vi "SwerveShortestTurnAlg.vi"(7 "Joystick Axes":dbl[](array[numeric]), 8 "SwerveMotorsFlipped?":bool, 9 "SwerveSpeed":dbl, 10 "AngleSetpoint":dbl, 11 "AngleEncoder":dbl) -> (2 "FlipSwerveMotors":bool, 3 "PIDInput":dbl)   [LabVIEW 2018]
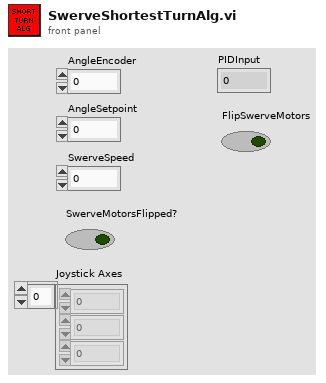
[diagram p1: front panel]
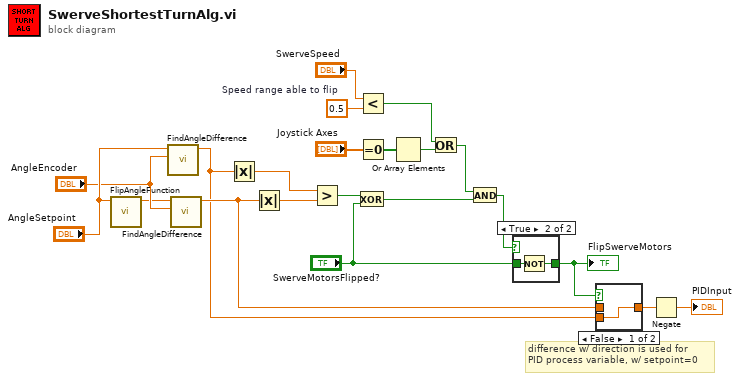
[diagram p0: block diagram]
diagram:
  w13 = 0.5  # Speed range able to flip
  # "difference w/ direction is used for\nPID process variable, w/ setpoint=0"
  n1 = call "FlipAngleFunction.vi"("AngleInput"="AngleSetpoint") -> ("AngleFlipped"=w15:dbl)  [unwired: 10 in]
  n2 = call "FindAngleDifference.vi"("AngleEncoder"="AngleEncoder", "AngleSetpoint"="AngleSetpoint") -> ("Distance/DirectionOfTurn"=w14:dbl)  [unwired: 9 in]
  n3 = call "FindAngleDifference.vi"("AngleEncoder"="AngleEncoder", "AngleSetpoint"=w15) -> ("Distance/DirectionOfTurn"=w16:dbl)  [unwired: 9 in]
  n4 = Absolute Value(x=w14) -> (abs(x)=w9:dbl)
  n5 = Absolute Value(x=w16) -> (abs(x)=w8:dbl)
  n6 = Greater?(x=w9, y=w8) -> (0:w11:bool)
  n7 = Exclusive Or(1:"SwerveMotorsFlipped?", 2:w11) -> (0:w6:bool)
  n8 = Less?(x="SwerveSpeed", y=w13) -> (x < y?=w1:bool)
  n9 = Equal To 0?(x="Joystick Axes") -> (x = 0?=w7:bool[])
  n10 = Or Array Elements(Boolean array=w7) -> (logical OR=w3:bool)
  n11 = Or(x=w1, y=w3) -> (x .or. y?=w5:bool)
  n12 = And(x=w5, y=w6) -> (x .and. y?=w2:bool)
  n13 = case shown="True" w2 {
    tunnel: "SwerveMotorsFlipped?" -> [w22 w24]
    tunnel: [w22 w23] -> w18
    frame False {
    }
    frame True {
      n14 = Not(x=w24) -> (.not. x?=w23:bool)
    }
  }
  "FlipSwerveMotors" <- w18
  n15 = case shown="False" w18 {
    tunnel: w14 -> [w25 _]
    tunnel: w16 -> [_ w26]
    tunnel: [w25 w26] -> w17
    frame False {
    }
    frame True {
    }
  }
  n16 = Negate(x=w17) -> (-x=→"PIDInput":dbl)
